vi "SET_JOE_JOHNSON.vi"(10 "argv":string[](array[string]), 11 "args":u8) -> ()   [LabVIEW 2011]
uses:
  joe_johnson/joe_johnson_state.ctl
  <vilib>/Rock Robotics/WPI/DriverStation/WPI_DriverStationStatusErrorCache.ctl
  Auto_Conf.vi
panel:
  in  "StateMaps":cluster{"Name":string, "State":T1}[](array[cluster])=[{"Name"="fold", "State"=enum."fold"}, {"Name"="down", "State"=enum."down"}, {"Name"="up", "State"=enum."up"}, {"Name"="ramp", "State"=enum."ramp"}, {"Name"="bridge", "State"=enum."bridge_lift"}, {"Name"="ramp_stay", "State"=enum."ramp_stay"}]
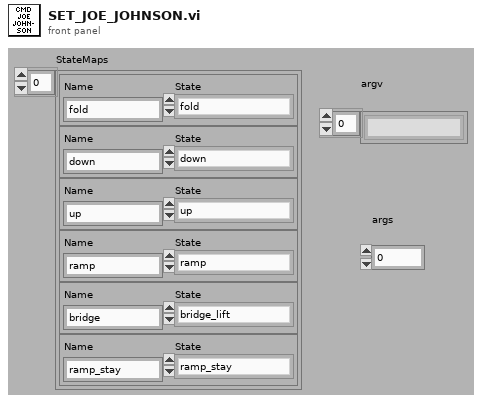
[diagram p1: front panel]
types:
  T1 = typedef "joe_johnson_state.ctl" = enum16{"fold", "down", "up", "ramp", "bridge_lift", "manual", "ramp_stay"}
  T2 = typedef "WPI_DriverStationStatusErrorCache.ctl" = enum16{"Get", "Set"}
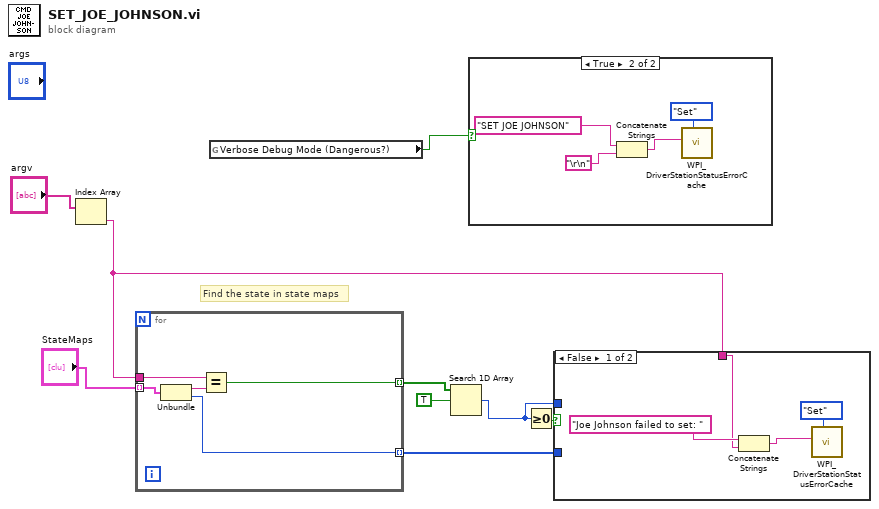
[diagram p0: block diagram]
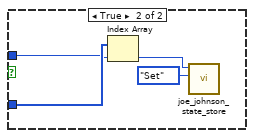
[diagram p3: hidden frame]
diagram:
  # "Find the state in state maps"
  n1 = Index Array(array="argv") -> (element=w2:string)  [unwired: 1 in]
  n2 = for {
    tunnel: w2 -> [w14]
    tunnel: "StateMaps" -> [w13] mode=indexing
    tunnel: [w11] -> w7 mode=indexing
    tunnel: [w10] -> w4 mode=indexing
    n3 = Unbundle(w13) -> ("Name"=w12:string, "State"=w10:T1)
    n4 = Equal?(x=w14, y=w12) -> (x = y?=w11:bool)
  }
  n5 = global read "Auto_Conf.vi" "Verbose Debug Mode (Dangerous?)"() -> (w1:bool)
  n6 = Search 1D Array(1D array=w7, element=TRUE) -> (index of element=w3:i32)  [unwired: 1 out]
  n7 = case shown="True" w1 {
    frame False {
    }
    frame True {
      n8 = Concatenate Strings("SET JOE JOHNSON" ("string"), "\r\n") -> (w16:string)
      n9 = call <vilib>:"WPI_DriverStationStatusErrorCache.vi"("StatusErrorCacheOp"=WPI_DriverStationStatusErrorCache."Set", "Error String"=w16) -> ()  [unwired: 10 out]
    }
  }
  n10 = Greater Or Equal To 0?(x=w3) -> (x >= 0?=w5:bool)
  n11 = case shown="False" w5 {
    tunnel: w4 -> [_ w26]
    tunnel: w3 -> [_ w25]
    tunnel: w2 -> [w19 _]
    frame False {
      n12 = Concatenate Strings("Joe Johnson failed to set: " ("string"), w19) -> (w20:string)
      n13 = call <vilib>:"WPI_DriverStationStatusErrorCache.vi"("StatusErrorCacheOp"=WPI_DriverStationStatusErrorCache."Set", "Error String"=w20) -> ()  [unwired: 10 out]
    }
    frame True {
      n14 = Index Array(array=w26, index=w25) -> (element=w24:T1)
      n15 = call "joe_johnson_state_store.vi"("data_store_mode"=enum16{"Set", "Get"}."Set", "joe_johnson_state"=w24) -> ()  [unwired: 7 in, 3 out]
    }
  }
